vi "Stop Button.vi"() -> ()   [LabVIEW 2020]
panel:
  out "Stop Ref":refnum<vi>
  in  "Stop Button":bool
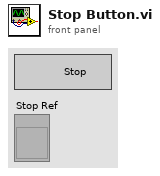
[diagram p1: front panel]
types:
  T1 = enum32{"Bad", "Idle", "Run top level", "Running"}
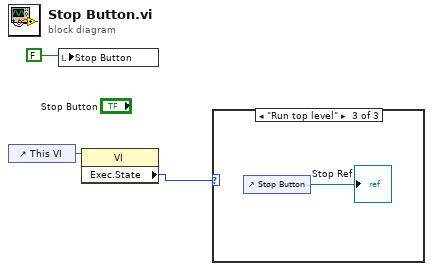
[diagram p0: block diagram]
diagram:
  n1 = control-ref of="This VI"() -> (w3:refnum<vi>)
  n2 = local write "Stop Button"(FALSE) -> ()
  n3 = property class="VI"(reference=w3) -> ("Exec.State"=w2:T1)  [unwired: 1 in, 2 out]
  n4 = case shown="\"Run top level\"" w2 {
    frame "Bad", Default {
    }
    frame "Idle" {
    }
    frame "Run top level" {
      n5 = control-ref of="Stop Button"() -> (→"Stop Ref":refnum<vi>)
    }
  }
